vi "Read Log.vi"(11 "log file path":string) -> (0 "error out":errorcluster, 3 "Response":string)   [LabVIEW 2020]
doc: "Returns the content of the log file located unter the log file path."
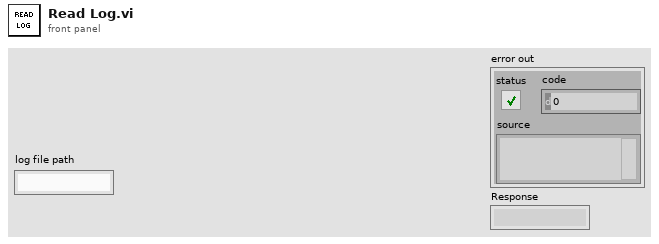
[diagram p1: front panel]
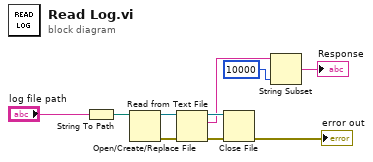
[diagram p0: block diagram]
diagram:
  n1 = String To Path(string="log file path") -> (path=w9:path)
  n2 = Open/Create/Replace File(file path (use dialog)=w9) -> (refnum out=w7:refnum<file>, error out=w8:errorcluster)  [unwired: 5 in, 1 out]
  n3 = Read from Text File(file (use dialog)=w7, error in=w8) -> (refnum out=w5:refnum<file>, text=w4:string, error out=w6:errorcluster)  [unwired: 2 in, 1 out]
  n4 = Close File(refnum=w5, error in=w6) -> (error out=→"error out":errorcluster)  [unwired: 1 out]
  n5 = String Subset(string=w4, length (rest)=10000 ("length (rest)")) -> (substring=→"Response":string)  [unwired: 1 in]
